vi "Varian Continuous.vi"(8 "error in":errorcluster, 10 "Varian Magnet.lvclass":refnum<class "Varian Magnet.lvclass">, 11 "Varian Continuous in":refnum<class "Varian Continuous.lvclass">) -> (0 "error out":errorcluster, 3 "Varian Continous out":refnum<class "Varian Continuous.lvclass">)   [LabVIEW 2009, in "Varian Continuous.lvclass"]
uses:
  Varian Continuous.lvclass
  Instruments/Varian Magnet/Varian Magnet.lvclass
  Scanner/Scanner.lvclass
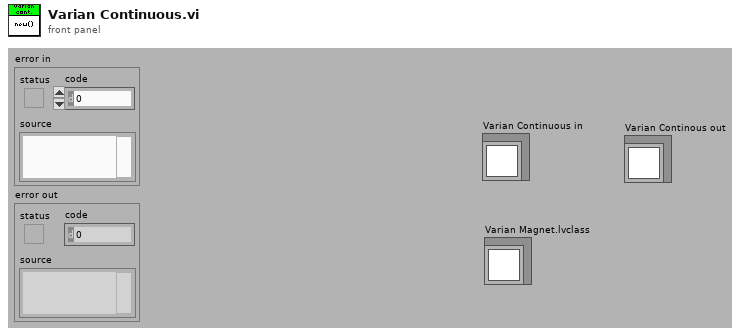
[diagram p1: front panel]
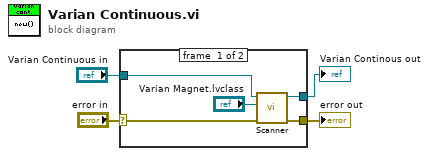
[diagram p0: block diagram]
diagram:
  n1 = case shown="No Error" "error in" {
    selector: "error in" -> [w6 w10]
    tunnel: "Varian Continuous in" -> [w9 w11]
    tunnel: [w8 w11] -> w2
    tunnel: [w5 w10] -> w1
    frame #0 {
      n2 = call "Scanner.vi"("error in (no error)"=w6, "Scannable"="Varian Magnet.lvclass", "Scanner.lvclass in"=w9) -> ("error out"=w5:errorcluster, "Scanner.lvclass out"=w8:refnum<class "Varian Continuous.lvclass">)  [unwired: 7 in]
    }
    frame #1 {
    }
  }
  "Varian Continous out" <- w2
  "error out" <- w1
